vi "kursory_1.vi"() -> ()   [LabVIEW 2013]
uses:
  <vilib>/measure/NI_MABase.lvlib
panel:
  out "Name":string
  in  "index":i32
  out "Char":i16
  in  "stop":bool
  in  "Array":T1(array[cluster]) {"amplitude" format="%0.2p"; "frequency" format="%0.2p"}
  out "Waveform Graph":waveform(dbl)[](graph)
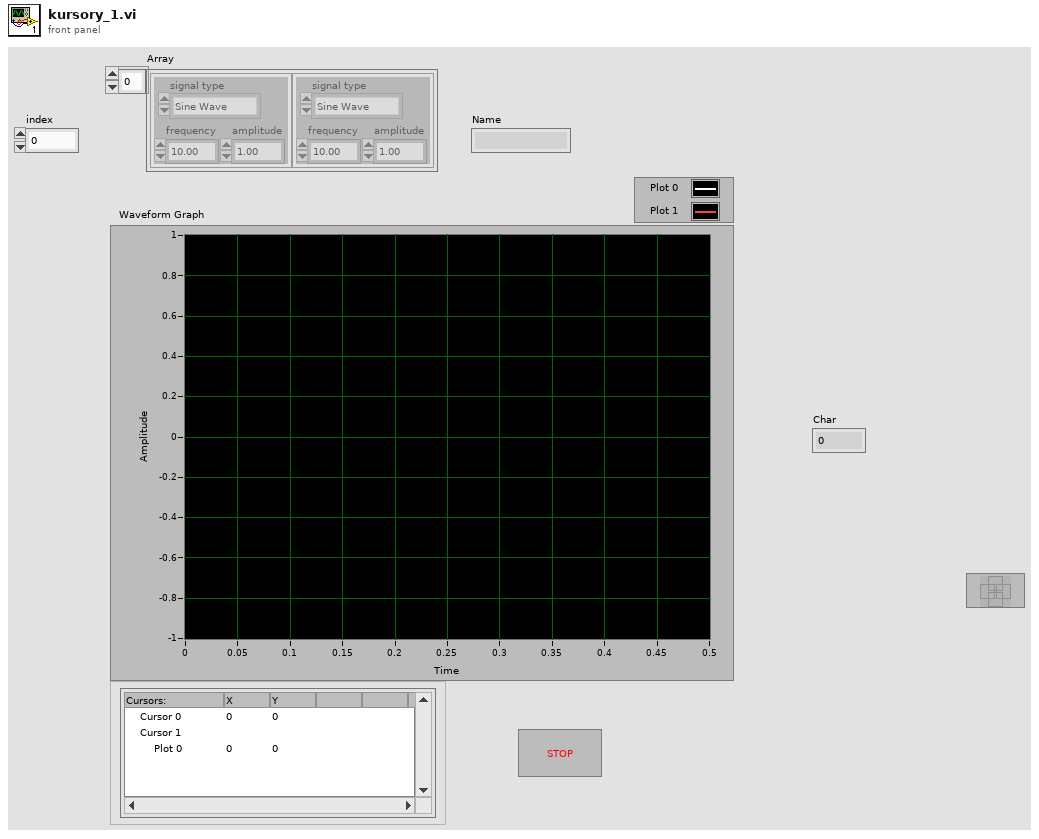
[diagram p1: front panel]
types:
  T1 = cluster{"signal type":enum16{"Sine Wave", "Triangle Wave", "Square Wave", "Sawtooth Wave"}, "frequency":dbl, "amplitude":dbl}[]
  T2 = enum16{"Sine Wave", "Triangle Wave", "Square Wave", "Sawtooth Wave"}
  T3 = typedef "LVCursorListTypeDef.ctl" = cluster{"Name":string, "Color":u32, "Style":u8, "Point Style":u8, "Name Visible":bool, "Allow Drag":bool, "Cursor Mode":u32, "Plot":i32, "Index":i32, "Position":cluster{"X":dbl, "Y":dbl}, "X Scale":u32, "Y Scale":u32, "Watch Plots":i32[], "Watch All Plots":bool, "Plot Area":i32, "Label Offset":cluster{"X":dbl, "Y":dbl}}[]
  T4 = cluster{"Name":string, "Color":u32, "Style":u8, "Point Style":u8, "Name Visible":bool, "Allow Drag":bool, "Cursor Mode":u32, "Plot":i32, "Index":i32, "Position":cluster{"X":dbl, "Y":dbl}, "X Scale":u32, "Y Scale":u32, "Watch Plots":i32[], "Watch All Plots":bool, "Plot Area":i32, "Label Offset":cluster{"X":dbl, "Y":dbl}}
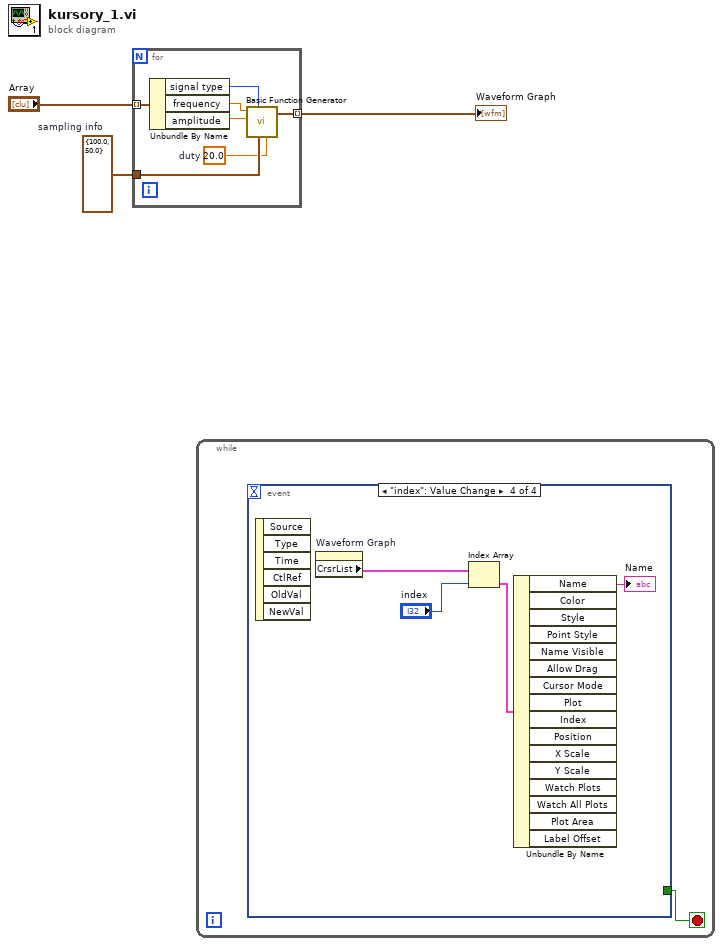
[diagram p0: block diagram]
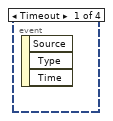
[diagram p2: hidden frame]
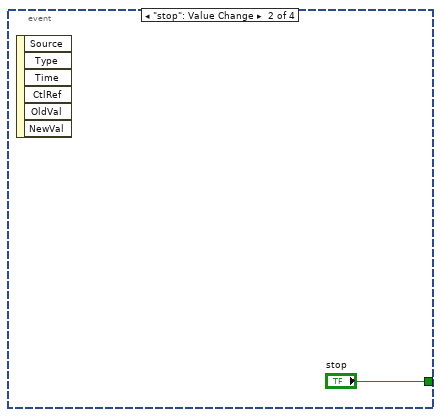
[diagram p3: hidden frame]
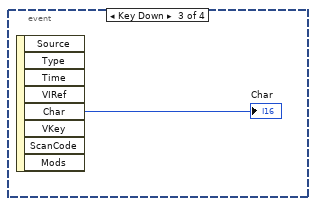
[diagram p4: hidden frame]
diagram:
  w3 = cluster{"Fs":dbl, "#s":dbl} {"Fs"=100.0, "#s"=50.0}  # sampling info
  n1 = for {
    tunnel: w3 -> [w10]
    tunnel: [w9] -> w2 mode=indexing
    tunnel: "Array" -> [w8] mode=indexing
    w4 = 20.0  # duty
    n2 = Unbundle By Name(w8) -> ("signal type"=w7:T2, "frequency"=w6:dbl, "amplitude"=w5:dbl)
    n3 = call <vilib>:"Basic Function Generator.vi"("square wave duty cycle (%)"=w4, "sampling info"=w10, "signal type"=w7, "amplitude"=w5, "frequency"=w6) -> ("signal out"=w9:waveform(dbl))  [unwired: 4 in, 2 out]
  }
  "Waveform Graph" <- w2
  n4 = while {
    stop <- w11 stop-if-true
    n5 = event shown="[3] \"index\": Value Change" {
      selector: _ -> [_ _ _ _]
      dyn-events: _ -> [_ _ _ _]
      timeout: _ -> [_ _ _ _]
      tunnel: [_ "stop" _ _] -> w11
      event Timeout {
        n6 = event-data() -> ()  [unwired: 1 in, 3 out]
      }
      event "stop": Value Change {
        n7 = event-data() -> ()  [unwired: 1 in, 6 out]
      }
      event Key Down {
        n8 = event-data() -> ("Char"=→"Char":i16)  [unwired: 1 in, 7 out]
      }
      event "index": Value Change {
        n9 = event-data() -> ()  [unwired: 1 in, 6 out]
        n10 = property on="Waveform Graph" class="WFGraph (strict)"() -> ("CrsrList"=w14:T3)  [unwired: 2 in, 2 out]
        n11 = Index Array(array=w14, index="index") -> (element=w15:T4)
        n12 = Unbundle By Name(w15) -> ("Name"=→"Name":string)  [unwired: 15 out]
      }
    }
  }
